vi "drive control (IO).vi"(1 "velocity":i16, 2 "drive vector":i8) -> ()   [LabVIEW 2009]
uses:
  <vilib>/eio/EIONode/EIONode.xnode
  <vilib>/rvi/eio/nirviEIOImplementation/nirviEIOImplementation.xnode
  <vilib>/rvi/eio/common/nirviEmuTemplateMethod_noerrors.vi
  <vilib>/rvi/eio/common/nirviEmuClasses.ctl
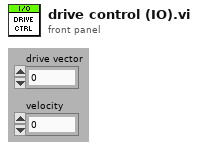
[diagram p1: front panel]
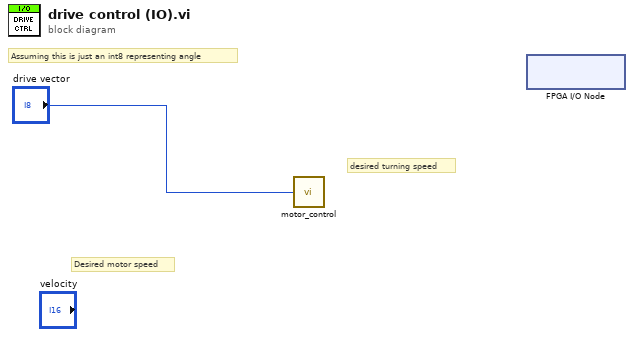
[diagram p0: block diagram]
diagram:
  # "desired turning speed"
  # "Desired motor speed"
  # "Assuming this is just an int8 representing angle"
  n1 = call "motor_control.vi"(0:"drive vector") -> (1:w1)  [unwired: 1 in]
  n2 = xnode "FPGA I/O Node"() -> ()  [unwired: 1 in, 2 out]
